vi "CreatingName_UsuallyInstrument.vi"(2 "error in (no error)":errorcluster, 3 "Name":string) -> (0 "error in (no error) 2":errorcluster, 1 "Output Name":string)   [LabVIEW 2019]
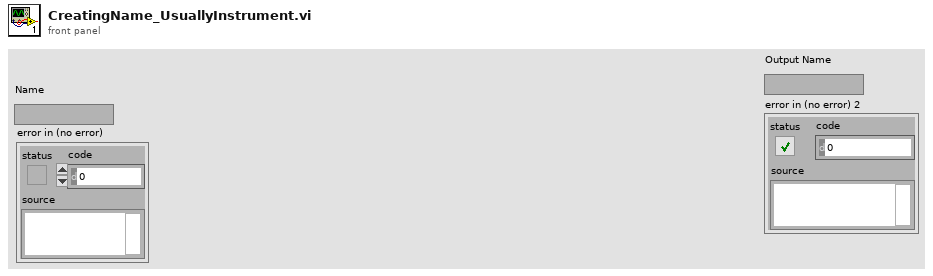
[diagram p1: front panel]
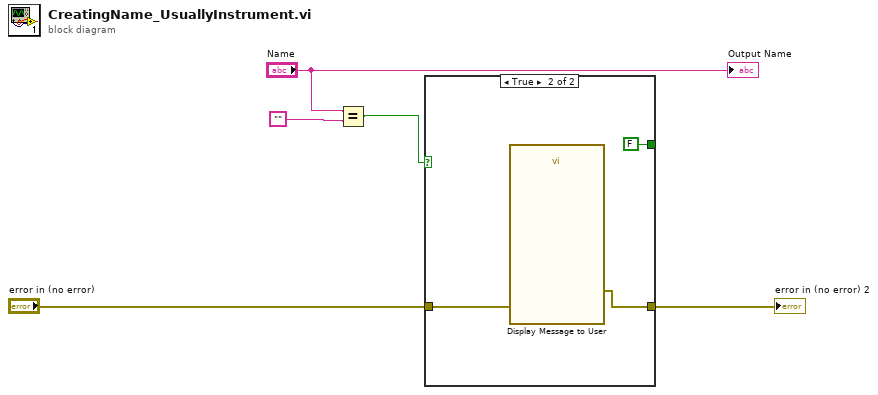
[diagram p0: block diagram]
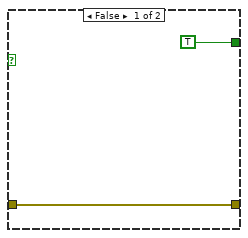
[diagram p2: hidden frame]
diagram:
  n1 = Equal?(x="Name", y="") -> (x = y?=w1:bool)
  n2 = case shown="True" w1 {
    tunnel: "error in (no error)" -> [w7 w10]
    tunnel: [w7 w9] -> w4
    tunnel: [TRUE FALSE] -> _
    frame False {
    }
    frame True {
      n3 = call "Display Message to User"("error in (no error)"=w10) -> ("error out"=w9:errorcluster)  [unwired: 9 in, 1 out]
    }
  }
  "error in (no error) 2" <- w4
  "Output Name" <- "Name"
